vi "testTwoServersSendEventsToClientsAtSameTime.vi"(8 "error in":errorcluster) -> (0 "error out":errorcluster)   [LabVIEW 2018]
uses:
  src/FactoryTcpServer/FactoryTcpServer.lvclass
  <vilib>/addons/_JKI Toolkits/Caraya/classes/Assert/Assert Equal Value_Variant.vi
  src/TcpServer/TcpServer.lvclass
  <vilib>/addons/_JKI Toolkits/Caraya/classes/Test/Test.lvclass
  <vilib>/addons/_JKI Toolkits/Caraya/classes/Assert/Assert.lvclass
panel:
  out "Run Server B error":errorcluster
  out "Run Server A error":errorcluster
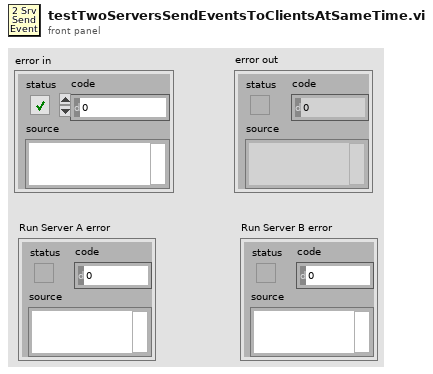
[diagram p1: front panel]
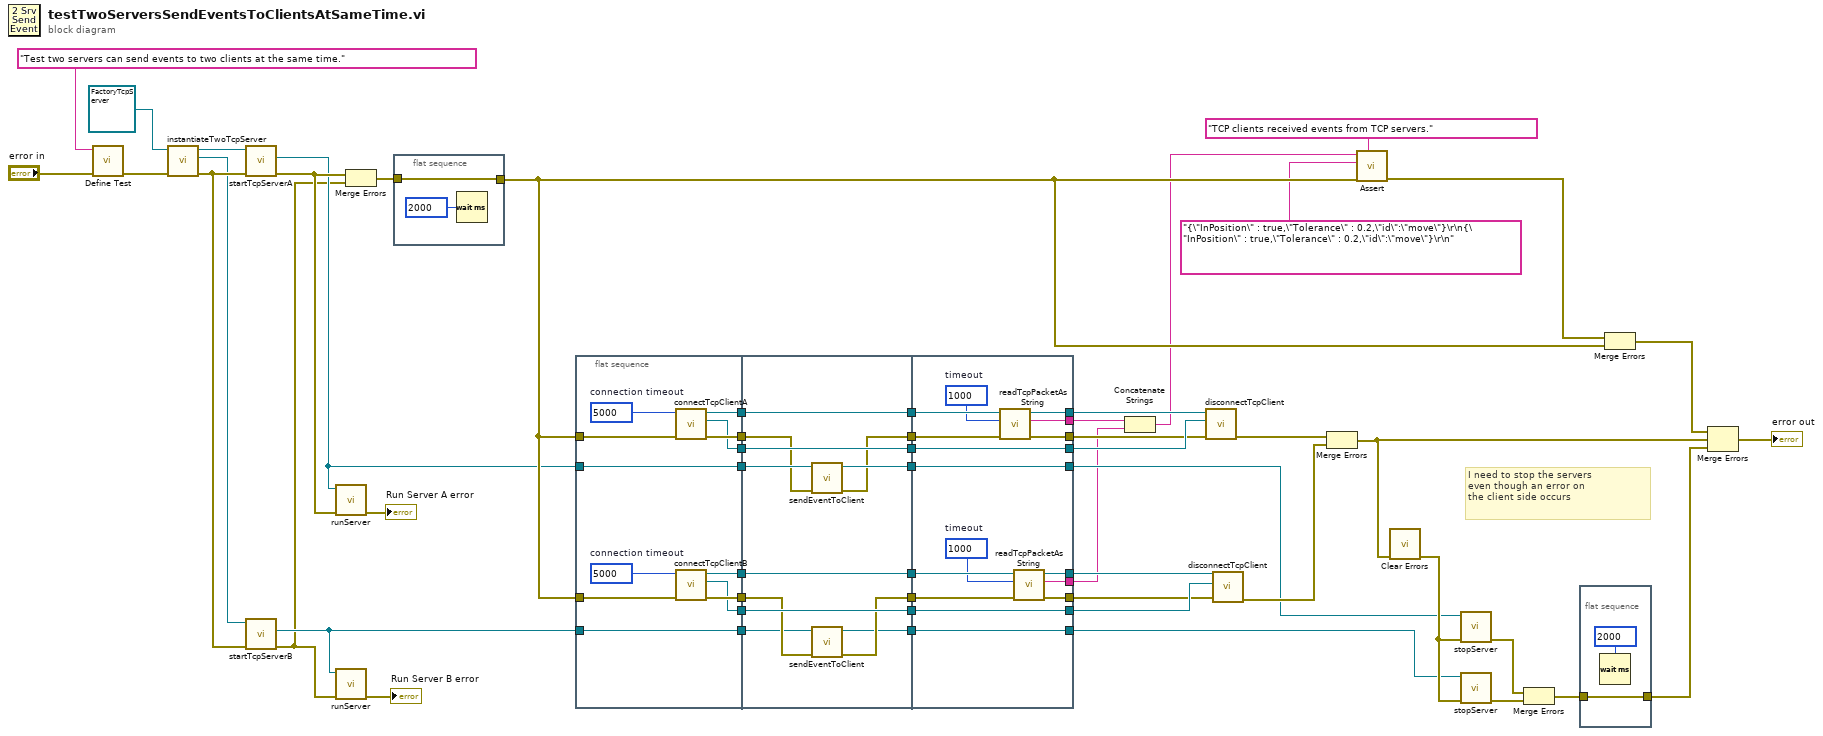
[diagram p0: block diagram]
diagram:
  # "I need to stop the servers \neven though an error on \nthe client side occurs"
  n1 = call <vilib>:"Define Test.vi"("error in (no error)"="error in", "Label (VI Title)"="Test two servers can send events to two clients at the same time.") -> ("error out"=w48:errorcluster)  [unwired: 9 in]
  n2 = call "instantiateTwoTcpServer.vi"("error in (no error)"=w48, "FactoryTcpServer in"=refnum<class "FactoryTcpServer.lvclass"> refnum) -> ("error out"=w4:errorcluster, "TcpServer 2 out"=w1:refnum<class "TcpServer.lvclass">, "TcpServer 1 out"=w2:refnum<class "TcpServer.lvclass">)  [unwired: 6 in, 1 out]
  n3 = call "startTcpServerA.vi"("error in (no error)"=w4, "TcpServer.lvclass"=w2) -> ("error out"=w43:errorcluster, "TcpServer out"=w39:refnum<class "TcpServer.lvclass">)  [unwired: 7 in, 1 out]
  n4 = call "startTcpServerB.vi"("error in (no error)"=w4, "TcpServer.lvclass"=w1) -> ("error out"=w5:errorcluster, "TcpServer out"=w34:refnum<class "TcpServer.lvclass">)  [unwired: 7 in, 1 out]
  n5 = call "runServer.vi"("error in (no error)"=w43, "TcpServer in"=w39) -> ("error out (no error)"=→"Run Server A error":errorcluster)  [unwired: 8 in, 1 out]
  n6 = call "runServer.vi"("error in (no error)"=w5, "TcpServer in"=w34) -> ("error out (no error)"=→"Run Server B error":errorcluster)  [unwired: 8 in, 1 out]
  n7 = Merge Errors(w43, w5) -> (w6:errorcluster)
  n8 = flat-sequence {
    tunnel: [w56] -> w40
    tunnel: w6 -> [w56]
    frame #0 {
      n9 = Wait (ms)(milliseconds to wait=u32 2000) -> ()  [unwired: 1 out]
    }
  }
  n10 = flat-sequence {
    tunnel: w40 -> [w69]
    tunnel: w40 -> [w68]
    tunnel: w39 -> [w67]
    tunnel: [w67] -> w38
    tunnel: [w66] -> w37
    tunnel: [w65] -> w36
    tunnel: [w64] -> w35
    tunnel: w34 -> [w64]
    tunnel: [w63] -> w33
    tunnel: [w62] -> w29
    tunnel: [w61] -> w21
    tunnel: [w60] -> w19
    tunnel: w38 -> [w78]
    tunnel: w37 -> [w76]
    tunnel: w36 -> [w73]
    tunnel: w35 -> [w71]
    tunnel: w33 -> [w74]
    tunnel: [w74] -> w32
    tunnel: [w75] -> w31
    tunnel: w29 -> [w81]
    tunnel: [w81] -> w27
    tunnel: [w77] -> w24
    tunnel: [w80] -> w22
    tunnel: w21 -> [w80]
    tunnel: [w79] -> w20
    tunnel: w19 -> [w79]
    tunnel: [w72] -> w18
    tunnel: [w70] -> w13
    tunnel: w32 -> [w97]
    tunnel: w31 -> [w96]
    tunnel: [w95] -> w30
    tunnel: [w94] -> w28
    tunnel: w27 -> [w94]
    tunnel: [w93] -> w26
    tunnel: [w92] -> w25
    tunnel: w24 -> [w92]
    tunnel: w22 -> [w91]
    tunnel: [w90] -> w16
    tunnel: w20 -> [w90]
    tunnel: w18 -> [w89]
    tunnel: [w88] -> w17
    tunnel: [w87] -> w15
    tunnel: [w86] -> w14
    tunnel: w13 -> [w86]
    tunnel: [w85] -> w9
    tunnel: [w84] -> w10
    frame #0 {
      w58 = 5000  # connection timeout
      w59 = 5000  # connection timeout
      n11 = call "connectTcpClientA.vi"("error in (no error)"=w68, "connection timeout (ms)"=w59) -> ("error out"=w66:errorcluster, "tel connection ID A out"=w62:refnum<k5>, "cmd connection ID A out"=w63:refnum<k5>)  [unwired: 7 in]
      n12 = call "connectTcpClientB.vi"("error in (no error)"=w69, "connection timeout (ms)"=w58) -> ("error out"=w65:errorcluster, "tel connection ID B out"=w60:refnum<k5>, "cmd connection ID B out"=w61:refnum<k5>)  [unwired: 7 in]
    }
    frame #1 {
      n13 = call "sendEventToClient.vi"("error in (no error)"=w76, "TcpServer out"=w78) -> ("error out"=w75:errorcluster, "tcpServer out"=w77:refnum<class "TcpServer.lvclass">)  [unwired: 8 in]
      n14 = call "sendEventToClient.vi"("error in (no error)"=w73, "TcpServer out"=w71) -> ("error out"=w72:errorcluster, "tcpServer out"=w70:refnum<class "TcpServer.lvclass">)  [unwired: 8 in]
    }
    frame #2 {
      w82 = 1000  # timeout
      w83 = 1000  # timeout
      n15 = call "readTcpPacketAsString.vi"("error in (no error)"=w96, "timeout ms (1000)"=w83, "connection ID in"=w97) -> ("error out"=w93:errorcluster, "TcpPacket"=w84:string, "connection ID out"=w95:refnum<k5>)  [unwired: 6 in]
      n16 = call "readTcpPacketAsString.vi"("error in (no error)"=w89, "timeout ms (1000)"=w82, "connection ID in"=w91) -> ("error out"=w87:errorcluster, "TcpPacket"=w85:string, "connection ID out"=w88:refnum<k5>)  [unwired: 6 in]
    }
  }
  n17 = Concatenate Strings(w10, w9) -> (w8:string)
  n18 = call "disconnectTcpClient.vi"("error in (no error)"=w26, "tel connection ID in"=w28, "cmd connection ID in"=w30) -> ("error out"=w49:errorcluster)  [unwired: 8 in]
  n19 = call "disconnectTcpClient.vi"("error in (no error)"=w15, "tel connection ID in"=w16, "cmd connection ID in"=w17) -> ("error out"=w47:errorcluster)  [unwired: 8 in]
  n20 = Merge Errors(w49, w47) -> (w45:errorcluster)
  n21 = call-poly <vilib>:"Assert.vi"("Label"="TCP clients received events from TCP servers.", "error in (no error)"=w40, "Y"="{\"InPosition\" : true,\"Tolerance\" : 0.2,\"id\":\"move\"}\r\n{\"InPosition\" : true,\"Tolerance\" : 0.2,\"id\":\"move\"}\r\n" ("concatenated string"), "X"=w8) -> ("error out"=w42:errorcluster)  [unwired: 7 in]
  n22 = call <vilib>:"Clear Errors.vi"("error in (no error)"=w45) -> ("error out"=w44:errorcluster)  [unwired: 5 in, 1 out]
  n23 = call "stopServer.vi"("error in (no error)"=w44, "tcpServer in"=w25) -> ("error out"=w53:errorcluster)  [unwired: 8 in, 1 out]
  n24 = call "stopServer.vi"("error in (no error)"=w44, "tcpServer in"=w14) -> ("error out"=w52:errorcluster)  [unwired: 8 in, 1 out]
  n25 = Merge Errors(w53, w52) -> (w51:errorcluster)
  n26 = flat-sequence {
    tunnel: w51 -> [w98]
    tunnel: [w98] -> w46
    frame #0 {
      n27 = Wait (ms)(milliseconds to wait=u32 2000) -> ()  [unwired: 1 out]
    }
  }
  n28 = Merge Errors(w42, w40) -> (w41:errorcluster)
  n29 = Merge Errors(w41, w45, w46) -> (→"error out":errorcluster)
